vi "Database-GetDBtime.vi"(1 "Idx":i32) -> (0 "DbTime":timestamp)   [LabVIEW 2016]
uses:
  Database.Global.vi
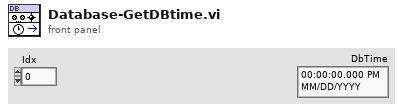
[diagram p1: front panel]
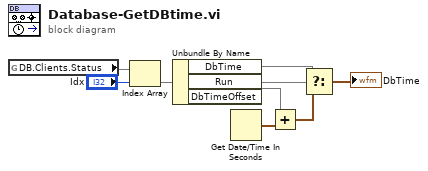
[diagram p0: block diagram]
diagram:
  n1 = global read "Database.Global.vi" "DB.Clients.Status"() -> (w7)
  n2 = Index Array(array=w7, index="Idx") -> (element=w5)
  n3 = Unbundle By Name(w5) -> ("DbTime"=w1, "Run"=w4, "DbTimeOffset"=w3)
  n4 = Get Date/Time In Seconds() -> (seconds since 1Jan1904=w8:timestamp)
  n5 = Add(x=w3, y=w8) -> (x+y=w2:timestamp)
  n6 = Select(t=w1, s=w4, f=w2) -> (s? t:f=→"DbTime":timestamp)
